vi "simple measure step.vi"(1 "apply measurement?":bool=TRUE, 5 "location":i16, 7 "state in":T1, 9 "num photons":u16) -> (8 "state out":T1)   [LabVIEW 2010]
uses:
  kalman simple pv state.ctl
  <vilib>/rvi/FXPMathLib/FxpSub/XNode/nifxpmath_Sub.xnode
  <vilib>/rvi/FXPMathLib/FxpSub/subVIs/nifxpmath_Sub_SimConfig.ctl
  <vilib>/fxp/LVFixedPointQuantizationPolicyTypeDef.ctl
  <vilib>/fxp/LVFixedPointOverflowPolicyTypeDef.ctl
  <vilib>/rvi/FXPMathLib/FxpMul/XNode/nifxpmath_Multiplier.xnode
  <vilib>/rvi/FXPMathLib/FxpMul/subVIs/nifxpmath_Mul_SimConfig.ctl
  <vilib>/rvi/FXPMathLib/FxpAdd/XNode/nifxpmath_Add.xnode
  <vilib>/rvi/FXPMathLib/FxpAdd/subVIs/nifxpmath_Add_SimConfig.ctl
  <vilib>/rvi/FXPMathLib/FxpSub/simVIs/DllFxpSubTemp_sub.vi
  <vilib>/rvi/FXPMathLib/FxpMul/simVIs/DllFxpMulTemp_sub.vi
  <vilib>/rvi/FXPMathLib/FxpAdd/simVIs/DllFxpAddTemp_sub.vi
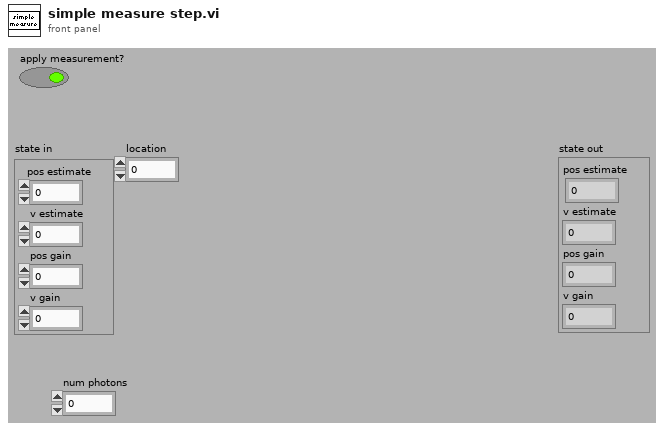
[diagram p1: front panel]
types:
  T1 = typedef "kalman simple pv state.ctl" = cluster{"pos estimate":fxp<+/-,32,16>, "v estimate":fxp<+/-,32,0>, "pos gain":fxp<+,32,0>, "v gain":fxp<+,32,0>}
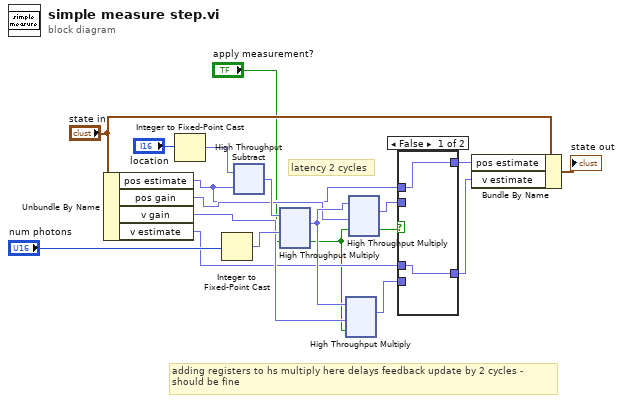
[diagram p0: block diagram]
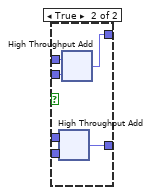
[diagram p2: hidden frame]
diagram:
  # "latency 2 cycles"
  # "adding registers to hs multiply here delays feedback update by 2 cycles - \nshould be fine"
  n1 = Unbundle By Name("state in") -> ("pos estimate"=w8:fxp<+/-,32,16>, "pos gain"=w11:fxp<+,32,0>, "v gain"=w10:fxp<+,32,0>, "v estimate"=w5:fxp<+/-,32,0>)
  n2 = Integer to Fixed-Point Cast(integer="location") -> (fixed-point=w16:fxp<+/-,16,16>)  [unwired: 1 in]
  n3 = Integer to Fixed-Point Cast(integer="num photons") -> (fixed-point=w13:fxp<+,16,16>)  [unwired: 1 in]
  n4 = xnode "High Throughput Subtract"("x"=w16, "y"=w8) -> ("x-y"=w14:fxp<+/-,32,16>)
  n5 = xnode "High Throughput Multiply"("x"=w14, "y"=w13, "input valid"="apply measurement?") -> ("x*y"=w12:fxp<+/-,32,16>, "output valid"=w2:bool)  [unwired: 1 in, 1 out]
  n6 = xnode "High Throughput Multiply"("x"=w12, "y"=w10, "input valid"=w2) -> ("x*y"=w6:fxp<+/-,32,0>)  [unwired: 1 in, 2 out]
  n7 = xnode "High Throughput Multiply"("x"=w12, "y"=w11, "input valid"=w2) -> ("x*y"=w9:fxp<+/-,32,16>, "output valid"=w1:bool)  [unwired: 1 in, 1 out]
  n8 = case shown="False" w1 {
    tunnel: w9 -> [_ w27]
    tunnel: w8 -> [w21 w26]
    tunnel: [w21 w25] -> w7
    tunnel: w6 -> [_ w24]
    tunnel: w5 -> [w20 w23]
    tunnel: [w20 w22] -> w4
    frame False {
    }
    frame True {
      n9 = xnode "High Throughput Add"("x"=w23, "y"=w24) -> ("x+y"=w22:fxp<+/-,32,0>)
      n10 = xnode "High Throughput Add"("x"=w26, "y"=w27) -> ("x+y"=w25:fxp<+/-,32,16>)
    }
  }
  n11 = Bundle By Name(cluster="state in", "pos estimate"=w7, "v estimate"=w4) -> (→"state out":T1)
